vi "Get Tree Item Name.vi"(8 "error in (no error)":errorcluster, 10 "Tag":string, 11 "TreeControl in":refnum<vi>) -> (0 "error out":errorcluster, 1 "Item Name":string, 2 "Tag out":string, 3 "TreeControl out":refnum<vi>)   [LabVIEW 2018]
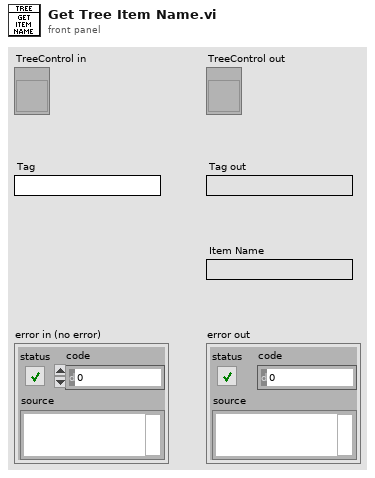
[diagram p1: front panel]
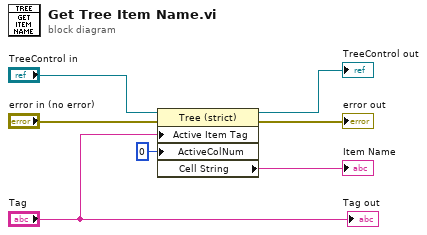
[diagram p0: block diagram]
diagram:
  n1 = property class="Tree (strict)"(reference="TreeControl in", error in="error in (no error)", "Active Item Tag"="Tag", "ActiveColNum"=0 ("Active Cell:Active Column Number")) -> (reference out=→"TreeControl out":refnum<vi>, error out=→"error out":errorcluster, "Cell String"=→"Item Name":string)
  "Tag out" <- "Tag"
